vi "PathPlanner_GeomUtil_RotationLerp.vi"(9 "T":dbl, 10 "EndVal":T1={"VALUE"=0.0, "COS"=1.0, "SIN"=0.0} {"SIN" format="%13.4f"; "COS" format="%13.4f"; "VALUE" format="%13.4f"}, 11 "StartVal":T1={"VALUE"=0.0, "COS"=1.0, "SIN"=0.0} {"SIN" format="%13.4f"; "COS" format="%13.4f"; "VALUE" format="%13.4f"}) -> (3 "Lerp":T1={"VALUE"=0.0, "COS"=1.0, "SIN"=0.0} {"SIN" format="%13.4f"; "COS" format="%13.4f"; "VALUE" format="%13.4f"})   [LabVIEW 2019, in "PathPlanner24.lvlib"]
uses:
  PathPlanner24.lvlib
  <vilib>/Rock Robotics/WPI/ThirdParty/JAS_Junk/TrajLib/TypeDef/ROTATION2D.ctl
  <vilib>/Rock Robotics/WPI/ThirdParty/JAS_Junk/TrajLib/Rotation2d_UnaryMinus.vi
  <vilib>/Rock Robotics/WPI/ThirdParty/JAS_Junk/TrajLib/Rotation2d_RotateBy.vi
  <vilib>/Rock Robotics/WPI/ThirdParty/JAS_Junk/TrajLib/Rotation2d_CreateAngle.vi
  <vilib>/Rock Robotics/WPI/ThirdParty/JAS_Junk/TrajLib/Rotation2d_CreateXY.vi
  <vilib>/Rock Robotics/WPI/ThirdParty/JAS_Junk/TrajLib/Util_CalcDist.vi
  <vilib>/Rock Robotics/WPI/ThirdParty/JAS_Junk/TrajLib/Trajectory_Library.lvlib
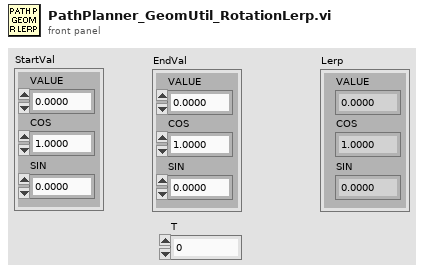
[diagram p1: front panel]
types:
  T1 = typedef "Trajectory_Library.lvlib/ROTATION2D.ctl" = cluster{"VALUE":dbl, "COS":dbl, "SIN":dbl}
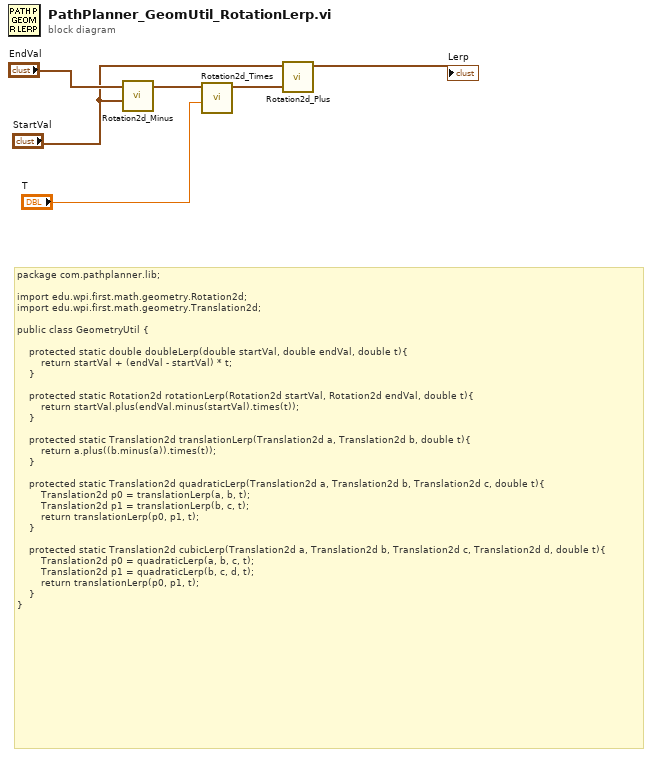
[diagram p0: block diagram]
diagram:
  # "package com.pathplanner.lib;\n\nimport edu.wpi.first.math.geometry.Rotation2d;\nimport edu.wpi.first.math.geometry.Translation2d;\n\npublic class GeometryUtil {\n\n    protected static double doubleLerp(double startVal, double endVal, double t){\n        return startVal + (endVal - startVal) * t;\n    }\n\n    protected static Rotation2d rotationLerp(Rotation2d startVal, Rotation2d endVal, double t){\n        return startVal.plus(endVal.minus(startVal).times(t));\n    }\n\n    protected static Translation2d translationLerp(Translation2d a, Translation2d b, double t){\n        return a.plus((b.minus(a)).times(t));\n    }\n\n    protected static Translation2d quadraticLerp(Translation2d a, Translation2d b, Translation2d c, double t){\n        Translation2d p0 = translationLerp(a, b, t);\n        Translation2d p1 = translationLerp(b, c, t);\n        return translationLerp(p0, p1, t);\n    }\n\n    protected static Translation2d cubicLerp(Translation2d a, Translation2d b, Translation2d c, Translation2d d, double t){\n        Translation2d p0 = quadraticLerp(a, b, c, t);\n        Translation2d p1 = quadraticLerp(b, c, d, t);\n        return translationLerp(p0, p1, t);\n    }\n}"
  n1 = call <vilib>:"Rotation2d_Minus.vi"("other ROTATION"="StartVal", "in ROTATION"="EndVal") -> ("out ROTATION"=w5:T1)  [unwired: 9 in]
  n2 = call <vilib>:"Rotation2d_Times.vi"("Scalar"="T", "in ROTATION"=w5) -> ("out ROTATION"=w3:T1)  [unwired: 9 in]
  n3 = call <vilib>:"Rotation2d_Plus.vi"("other ROTATION"=w3, "in ROTATION"="StartVal") -> ("out ROTATION"=→"Lerp":T1)  [unwired: 9 in]
